vi "Falling Edge True.vi"(11 "Input":bool) -> (3 "Output":bool)   [LabVIEW 2015]
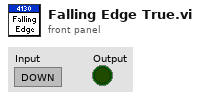
[diagram p1: front panel]
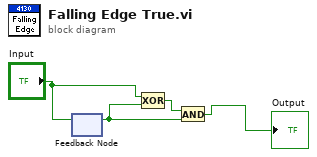
[diagram p0: block diagram]
diagram:
  n1 = feedback #1() -> (w3:bool)  [unwired: 1 in]
  n2 = feedback-in #1("Input") -> ()
  n3 = Compound Arithmetic op=XOR("Input", w3) -> (w2:bool)
  n4 = And(x=w2, y=w3) -> (x .and. y?=→"Output":bool)
